vi "Initialize Adpater Module.vi"(5 "Force Init":bool, 7 "Timeout (s)":dbl=5.0 caption="Time Target (s)", 8 "error in":errorcluster, 11 "FPGA VI Reference In":refnum<k20>) -> (0 "error out":errorcluster, 2 "FAM Configured":bool=TRUE, 3 "FPGA VI Reference Out":refnum<k20>)   [LabVIEW 2012, in "FlexRIO Host Library (User).lvlib"]
doc: "This VI initializes adpater mddule"
uses:
  <userlib>/FlexRIO Host Library/FlexRIO Host Library (User).lvlib
  <vilib>/rvi/errors/niLvFpgaAdjustHostInterfaceError.vi
  <vilib>/LabVIEW Targets/FPGA/FlexRIO/CustomFPGAMethods/79XXR_Method_IOModuleStatusImpl.vi
  <vilib>/rvi/interface/nirviReadWriteControl/nirviReadWriteControl.xnode
  <vilib>/rvi/interface/nirviMethod/nirviMethod.xnode
  NiFpgaLv.dll
  <vilib>/rvi/interface/Simulation/niFpgaSimulationCallBeginRW.vi
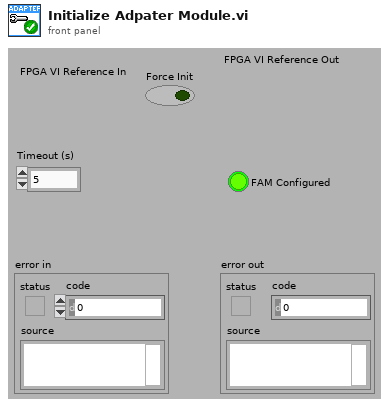
[diagram p1: front panel]
types:
  T1 = cluster{"io mod.initialization done":bool, "io mod.configuration error":bool, "io mod.synthesizer locked":bool, "io mod.spi idle":bool}
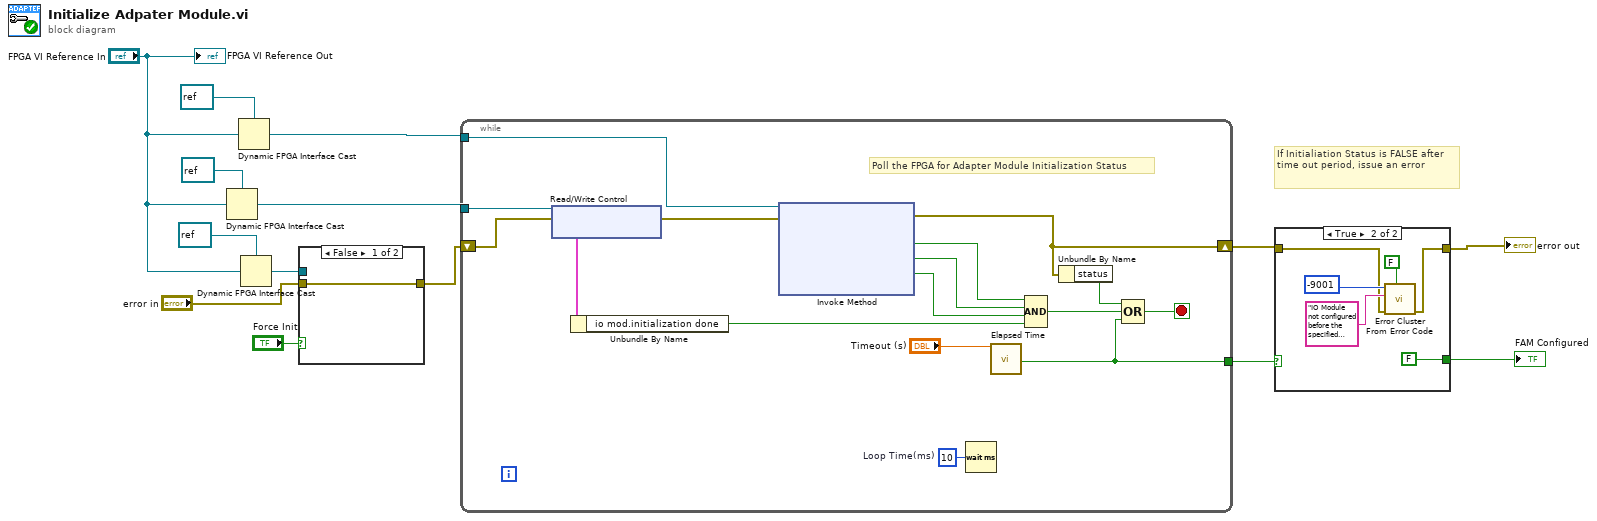
[diagram p0: block diagram]
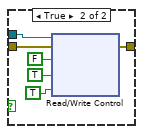
[diagram p2: hidden frame]
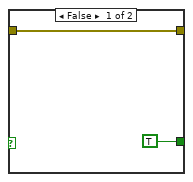
[diagram p3: hidden frame]
diagram:
  # "If Initialiation Status is FALSE after time out period, issue an error"
  n1 = Dynamic FPGA Interface Cast(Session In=refnum<k20> refnum ("Type"), Type="FPGA VI Reference In") -> (Session Out=w10:refnum<k20>)
  n2 = Dynamic FPGA Interface Cast(Session In=refnum<k20> refnum ("Type"), Type="FPGA VI Reference In") -> (Session Out=w7:refnum<k20>)
  n3 = Dynamic FPGA Interface Cast(Session In=refnum<k20> refnum ("Type"), Type="FPGA VI Reference In") -> (Session Out=w5:refnum<k20>)
  n4 = case shown="False" "Force Init" {
    tunnel: w5 -> [_ w21]
    tunnel: "error in" -> [w15 w20]
    tunnel: [w15 w19] -> w3
    frame False {
    }
    frame True {
      n5 = xnode "Read/Write Control"("FPGA VI Reference In"=w21, "error in"=w20, "Force Init"=FALSE, "Force Init"=TRUE, "Force Init"=TRUE) -> ("error out"=w19:errorcluster)  [unwired: 1 out]
    }
  }
  n6 = while {
    shift-right: [w32] -> w14
    shift-left: w3 -> [w25]
    tunnel: [w33] -> w13
    tunnel: w10 -> [w26]
    tunnel: w7 -> [w22]
    stop <- w36 stop-if-true
    w37 = u32 10  # Loop Time(ms)
    # "Poll the FPGA for Adapter Module Initialization Status"
    n7 = xnode "Read/Write Control"("FPGA VI Reference In"=w26, "error in"=w25) -> ("error out"=w24:errorcluster, "IO Module Status"=w23:T1)  [unwired: 1 out]
    n8 = Unbundle By Name(w23) -> ("io mod.initialization done"=w27:bool)
    n9 = xnode "Invoke Method"("FPGA VI Reference In"=w22, "error in"=w24) -> ("error out"=w32:errorcluster, "IO Module Present?"=w30:bool, "Power Enabled?"=w29:bool, "IO Enabled?"=w28:bool)  [unwired: 2 out]
    n10 = Wait (ms)(milliseconds to wait=w37) -> ()  [unwired: 1 out]
    n11 = call "Elapsed Time"("Time Target (s)"="Timeout (s)") -> ("Time has Elapsed"=w33:bool)  [unwired: 11 in, 7 out]
    n12 = Compound Arithmetic op=AND(w30, w29, w28, w27) -> (w31:bool)
    n13 = Unbundle By Name(w32) -> ("status"=w35:bool)
    n14 = Compound Arithmetic op=OR(w35, w31, w33) -> (w36:bool)
  }
  n15 = case shown="True" w13 {
    tunnel: w14 -> [w39 w41]
    tunnel: [w39 w44] -> w12
    tunnel: [TRUE ("Master FAM Configured") FALSE ("Master FAM Configured")] -> w11
    frame False {
    }
    frame True {
      n16 = call <vilib>:"Error Cluster From Error Code.vi"("show call chain? (False)"=FALSE, "error in (no error)"=w41, "error message (\"\")"="IO Module not configured before the specified timeout." ("source"), "error code (0)"=-9001 ("code")) -> ("error out"=w44:errorcluster)  [unwired: 5 in]
    }
  }
  "error out" <- w12
  "FAM Configured" <- w11
  "FPGA VI Reference Out" <- "FPGA VI Reference In"
